vi "RT_Main.vi"() -> ()   [LabVIEW 2014]
uses:
  <vilib>/rvi/interface/nirviOpenFPGA/nirviOpenFPGA.xnode
  <vilib>/rvi/interface/nirviMethod/nirviMethod.xnode
  <vilib>/FPGAPlugInAG/Dynamic/niLvFpga_ReadFifo_Dynamic.vi
  <vilib>/rvi/errors/niLvFpgaMergeErrorWithErrorCode.vi
panel:
  out "temp":dbl[](array[numeric])
  out "Data":i16[](array[numeric])
  out "Elements Remaining":u32
  in  "stop":bool
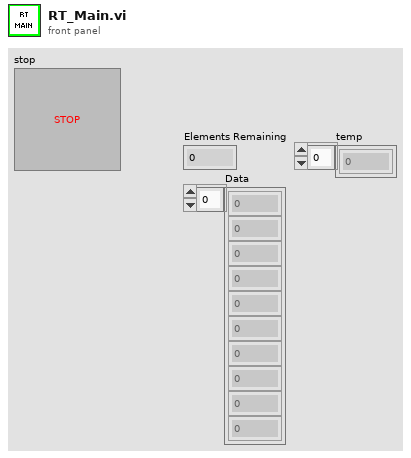
[diagram p1: front panel]
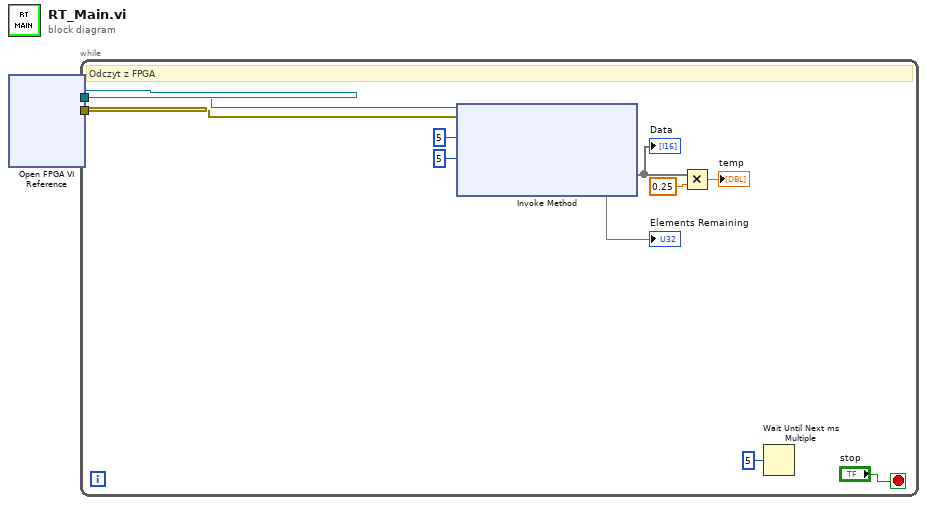
[diagram p0: block diagram]
diagram:
  n1 = xnode "Open FPGA VI Reference"() -> ("FPGA VI Reference Out"=w2:refnum<k20>, "error out"=w1:errorcluster)  [unwired: 2 in]
  n2 = while {
    tunnel: w2 -> [w4]
    tunnel: w1 -> [w3]
    stop <- "stop" stop-if-true
    # "Odczyt z FPGA"
    n3 = xnode "Invoke Method"("FPGA VI Reference In"=w4, "error in"=w3, "Number of Elements"=u32 5, "Timeout (ms)"=5) -> ("Data"=w7:void[], "Elements Remaining"=→"Elements Remaining")  [unwired: 2 out]
    "Data" <- w7
    n4 = Multiply(x=w7, y=0.25) -> (x*y=→"temp":dbl)
    n5 = Wait Until Next ms Multiple(millisecond multiple=u32 5) -> ()  [unwired: 1 out]
  }
